vi "pi_coef_conv.vi"(11 "PI Control input":T1) -> (3 "PI Control output":T1)   [LabVIEW 2015, in "Hardware.lvlib"]
uses:
  Hardware.lvlib
  PI Compensator.ctl
  Settings/Settings.lvlib
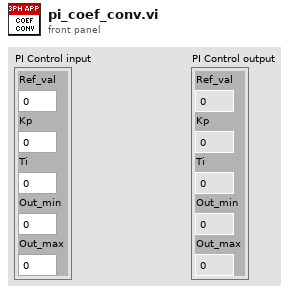
[diagram p1: front panel]
types:
  T1 = typedef "Settings.lvlib/PI Compensator.ctl" = cluster{"Ref_val":sgl, "Kp":sgl, "Ti":sgl, "Out_min":sgl, "Out_max":sgl}
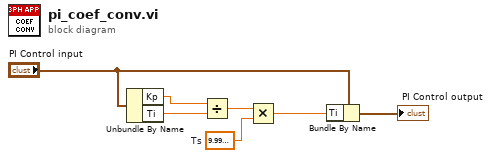
[diagram p0: block diagram]
diagram:
  w2 = sgl 1e-05  # Ts
  n1 = Unbundle By Name("PI Control input") -> ("Kp"=w4:sgl, "Ti"=w5:sgl)
  n2 = Divide(x=w4, y=w5) -> (x/y=w3:sgl)
  n3 = Multiply(x=w3, y=w2) -> (x*y=w1:sgl)
  n4 = Bundle By Name(cluster="PI Control input", "Ti"=w1) -> (→"PI Control output":T1)
